vi "Control_Panel_정리.vi"() -> ()   [LabVIEW 2014]
panel:
  in  "COM Port":string
  in  "Dump":dbl[](array[numeric])
  out "Connected":bool
  in  "Start":bool
  out "Communication Stopped":bool
  out "Acquisition Mode":bool
  out "Device Control Enabled":bool
  in  "Value Achieving Status":string
  in  "Connection":string
  in  "Enable Blink Detection Err Code":string
  in  "Write DataLog Path":string
  in  "Set Data Log Path":string
  in  "Connection ID":string
  in  "선택된 기능":string="응급"
  in  "전체종료 여부":string
  in  "Brain":path
  in  "ERP_Parameters_of_NonTarget_prior":path=path "C:/Emotion_Research/MyungjooWon_Training_Test(LDA)/2014-06-19/ERP_Parameters_of_NonTarget_prior.txt"
  in  "ERP_Parameters_of_Target_prior":path=path "C:/Emotion_Research/MyungjooWon_Training_Test(LDA)/2014-06-19/ERP_Parameters_of_Target_prior.txt"
  in  "Maximum_Iteration":i64=100
  in  "in":path=path "C:/Emotion_Research/MyungjooWon_Training_Test(LDA)/2014-06-19/in_SWLDA.txt"
  in  "Fatigue_Threshold":path
  in  "EEG_Channel_Num":i32=1
  in  "rate":dbl=512.0 caption="Rate" format="%0.2f"
  in  "sample mode":i32(ring)=10123 items=["유한 샘플"=10178, "연속 샘플"=10123, "하드웨어 타이밍에 의한 단일 포인트"=12522]
  in  "input terminal configuration":i32(ring)=10078 items=["기본값"=-1, "RSE"=10083, "NRSE"=10078, "차동"=10106, "유사 차동"=12529]
  in  "physical channels":tag="cDAQ1Mod5/ai0:6"
  in  "Experimentation_num":i32=2
  in  "LDA_Matrix":path=path "C:/Emotion_Research/MyungjooWon_Training_Test(LDA)/2014-06-19/LDA_Matrix_Value_SWLDA.txt"
  in  "피험자 이름":string="MyungjooWon"
  in  "정지":bool
  in  "Frame Length":i32=20
  in  "Flash_Repeat":i32=20
  in  "Random_num":i32=6
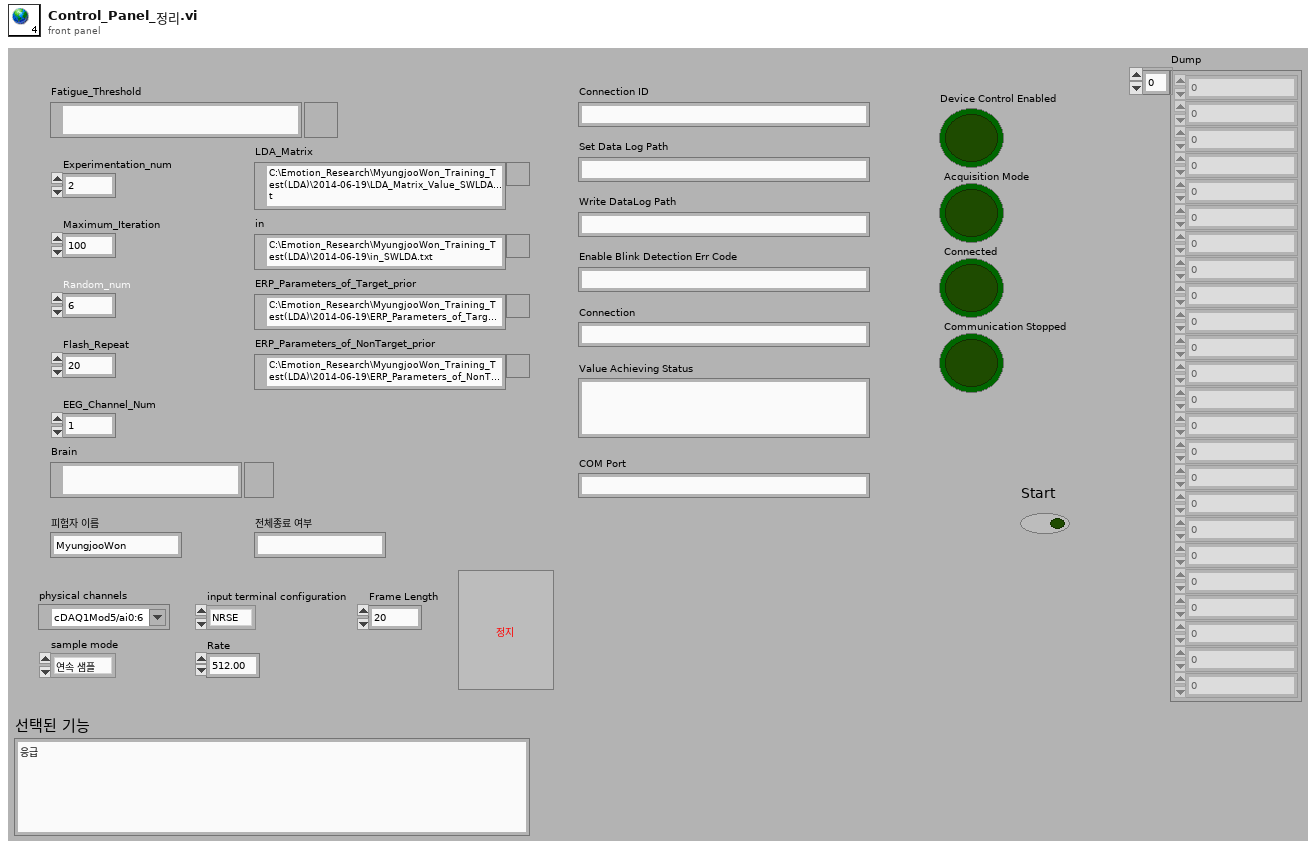
[diagram p1: front panel]
diagram:
